vi "UIStep Execte UI Init.vi"(9 "Project Path":path, 10 "UI Setting":T1={"Embedded"=FALSE, "Size"=enum."Small", "Title"="", "Content"="", "Text Style"={"Font"="", "Size"=0.0, "Justification"=1, "TextColor"=0, "BGColor"=0, "Bold"=FALSE}, "Buttons"={"Button1"={"Label"="", "Size"=0.0, "TextColor"=0, "BGColor"=0, "Bold"=FALSE}, "Button2"={"Label"="", "Size"=0.0, "TextColor"=0, "BGColor"=0, "Bold"=FALSE}}, "Image"=path "", "Enable Input"=FALSE, "Input Validation"=""} {"Text Style"."Justification" items=["Left", "Center", "Right"]}, 11 "UI Control":T2) -> (3 "UI Control out":T2)   [LabVIEW 2015, in "UIStep.lvclass"]
uses:
  UIStep.lvclass
  <vilib>/Utility/miscctls.llb/LVPointTypeDef.ctl
  <vilib>/Utility/miscctls.llb/LVRectTypeDef.ctl
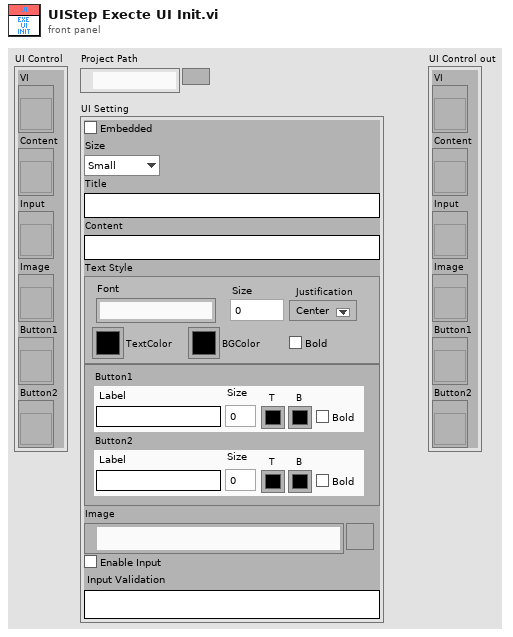
[diagram p1: front panel]
types:
  T1 = cluster{"Embedded":bool, "Size":enum16{"Small", "Middle", "Big"}, "Title":string, "Content":string, "Text Style":cluster{"Font":string, "Size":dbl, "Justification":u16, "TextColor":u32, "BGColor":u32, "Bold":bool}, "Buttons":cluster{"Button1":cluster{"Label":string, "Size":dbl, "TextColor":u32, "BGColor":u32, "Bold":bool}, "Button2":cluster{"Label":string, "Size":dbl, "TextColor":u32, "BGColor":u32, "Bold":bool}}, "Image":path, "Enable Input":bool, "Input Validation":string}
  T2 = cluster{"VI":refnum<vi>, "Content":refnum<vi>, "Input":refnum<vi>, "Image":refnum<vi>, "Button1":refnum<vi>, "Button2":refnum<vi>}
  T3 = typedef "LVPointTypeDef.ctl" = cluster{"Horizontal":i16, "Vertical":i16}
  T4 = cluster{"Label":string, "Size":dbl, "TextColor":u32, "BGColor":u32, "Bold":bool}
  T5 = cluster{"Font":string, "Size":dbl, "Justification":u16, "TextColor":u32, "BGColor":u32, "Bold":bool}
  T6 = typedef "imagedata.ctl" = cluster{"image type":i32, "image depth":i32, "image":u8[], "mask":u8[], "colors":u32[], "Rectangle":cluster{"left":i16, "top":i16, "right":i16, "bottom":i16}}
  T7 = typedef "LVRectTypeDef.ctl" = cluster{"Left":i16, "Top":i16, "Right":i16, "Bottom":i16}
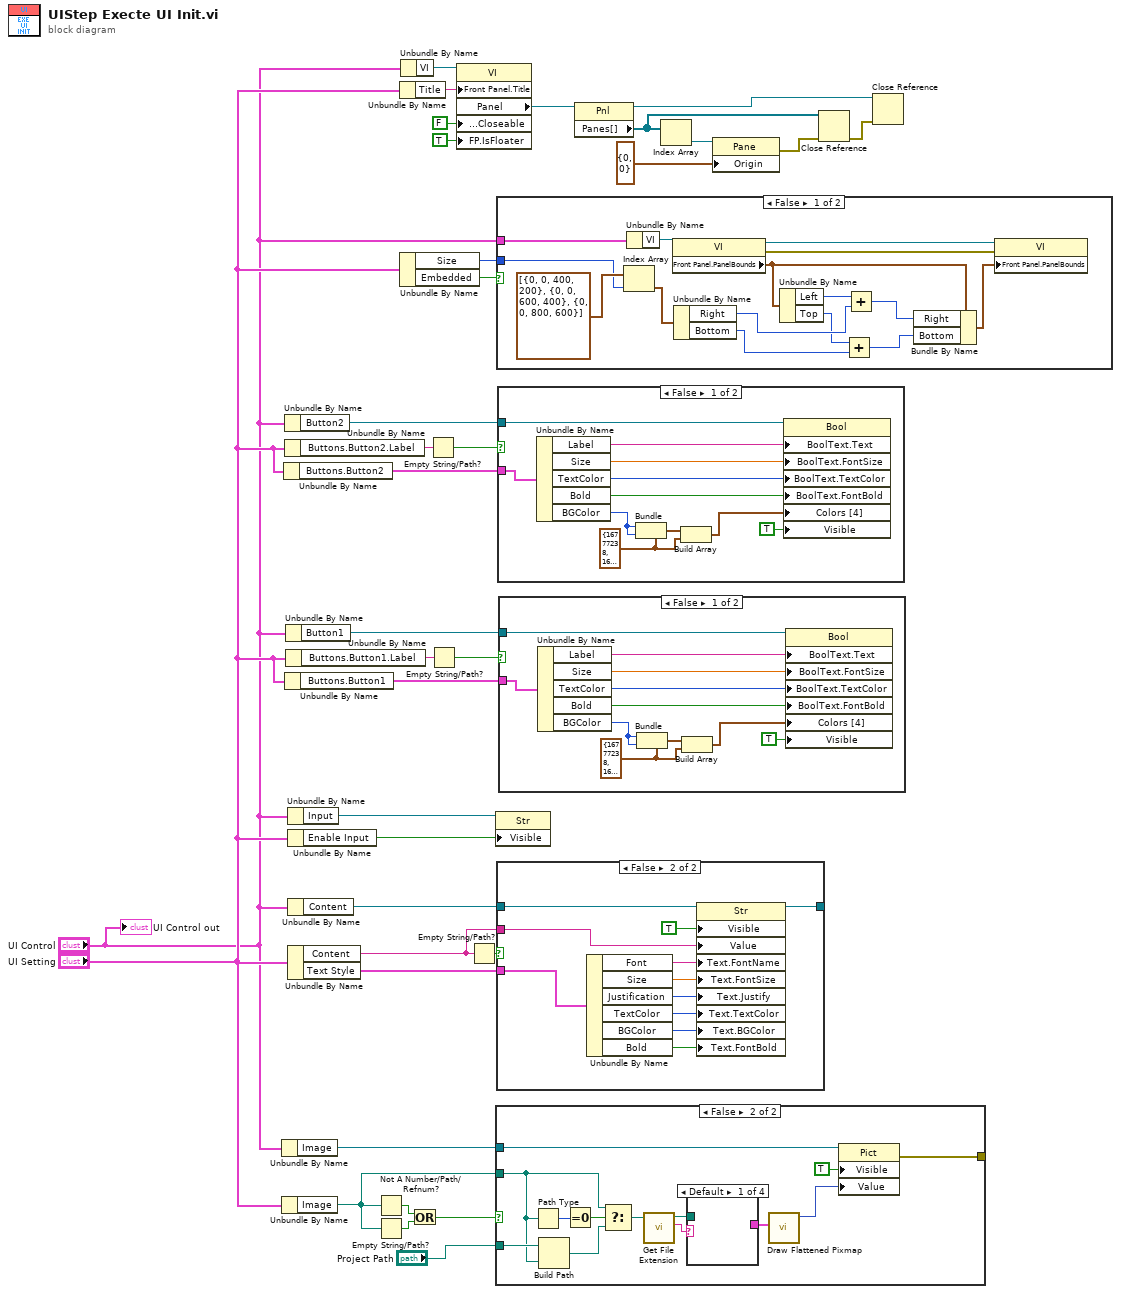
[diagram p0: block diagram]
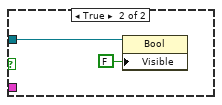
[diagram p3: hidden frame]
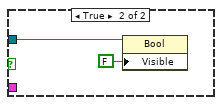
[diagram p4: hidden frame]
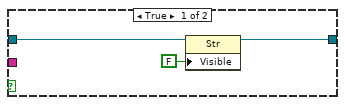
[diagram p5: hidden frame]
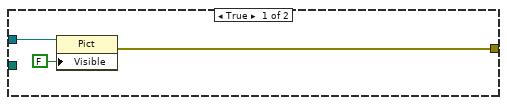
[diagram p6: hidden frame]
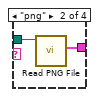
[diagram p7: hidden frame]
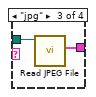
[diagram p8: hidden frame]
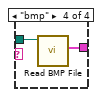
[diagram p9: hidden frame]
diagram:
  n1 = Unbundle By Name("UI Control") -> ("Image"=w35:refnum<vi>)
  n2 = Unbundle By Name("UI Setting") -> ("Image"=w31:path)
  n3 = Unbundle By Name("UI Setting") -> ("Buttons.Button2"=w20:T4)
  n4 = Unbundle By Name("UI Control") -> ("Button2"=w19:refnum<vi>)
  n5 = Unbundle By Name("UI Setting") -> ("Buttons.Button2.Label"=w17:string)
  n6 = Unbundle By Name("UI Setting") -> ("Buttons.Button1"=w21:T4)
  n7 = Unbundle By Name("UI Control") -> ("Button1"=w22:refnum<vi>)
  n8 = Unbundle By Name("UI Setting") -> ("Buttons.Button1.Label"=w24:string)
  n9 = Unbundle By Name("UI Control") -> ("Input"=w25:refnum<vi>)
  n10 = Unbundle By Name("UI Setting") -> ("Enable Input"=w3:bool)
  n11 = Unbundle By Name("UI Control") -> ("Content"=w28:refnum<vi>)
  n12 = Unbundle By Name("UI Setting") -> ("Content"=w26:string, "Text Style"=w27:T5)
  n13 = Not A Number/Path/Refnum?(number/path/refnum=w31) -> (NaN/Path/Refnum?=w33:bool)
  n14 = Empty String/Path?(string/path=w31) -> (empty?=w34:bool)
  n15 = Unbundle By Name("UI Setting") -> ("Title"=w15:string)
  n16 = Unbundle By Name("UI Setting") -> ("Size"=w6:enum16{"Small", "Middle", "Big"}, "Embedded"=w7:bool)
  n17 = Unbundle By Name("UI Control") -> ("VI"=w16:refnum<vi>)
  n18 = Or(x=w33, y=w34) -> (x .or. y?=w32:bool)
  n19 = Empty String/Path?(string/path=w17) -> (empty?=w18:bool)
  n20 = Empty String/Path?(string/path=w24) -> (empty?=w23:bool)
  n21 = property class="VI"(reference=w16, "Front Panel.Title"=w15, "Front Panel.Closeable"=FALSE ("Front Panel Window:Closeable"), "FP.IsFloater"=TRUE ("Front Panel Window:Is Floating")) -> ("Panel"=w14:refnum<vi>)  [unwired: 1 in, 2 out]
  n22 = Empty String/Path?(string/path=w26) -> (empty?=w29:bool)
  n23 = property class="Str"(reference=w25, "Visible"=w3) -> ()  [unwired: 1 in, 2 out]
  n24 = case shown="False" w32 {
    tunnel: w35 -> [w38 w51]
    tunnel: w31 -> [_ w46]
    tunnel: "Project Path" -> [_ w47]
    tunnel: [w36 w42] -> _
    frame True {
      n25 = property class="Pict"(reference=w38, "Visible"=FALSE) -> (error out=w36:errorcluster)  [unwired: 1 in, 1 out]
    }
    frame False {
      n26 = Path Type(1:w46) -> (0:w49:i16)
      n27 = Build Path(base path=w47, name or relative path=w46) -> (appended path=w45:path)
      n28 = Equal To 0?(x=w49) -> (x = 0?=w48:bool)
      n29 = Select(t=w46, s=w48, f=w45) -> (s? t:f=w41:path)
      n30 = call <vilib>:"Get File Extension.vi"("file"=w41) -> ("lowercase file extension"=w39:string, "dup file"=w40:path)  [unwired: 6 in, 3 out]
      n31 = case shown="Default" w39 {
        tunnel: [_ w53 w55 w57] -> w44
        tunnel: w40 -> [_ w52 w54 w56]
        frame Default {
        }
        frame "png" {
          n32 = call <vilib>:"Read PNG File.vi"("path to PNG file"=w52) -> ("image data"=w53:T6)  [unwired: 8 in, 2 out]
        }
        frame "jpg" {
          n33 = call <vilib>:"Read JPEG File.vi"("path to JPEG file"=w54) -> ("image data"=w55:T6)  [unwired: 8 in, 2 out]
        }
        frame "bmp" {
          n34 = call <vilib>:"Read BMP File.vi"("path to BMP file"=w56) -> ("image data"=w57:T6)  [unwired: 8 in, 2 out]
        }
      }
      n35 = call <vilib>:"Draw Flattened Pixmap.vi"("image data"=w44) -> ("new picture"=w43:picture)  [unwired: 8 in]
      n36 = property class="Pict"(reference=w51, "Visible"=TRUE, "Value"=w43) -> (error out=w42:errorcluster)  [unwired: 1 in, 1 out]
    }
  }
  n37 = case shown="False" w7 {
    tunnel: "UI Control" -> [w71 _]
    tunnel: w6 -> [w69 _]
    frame False {
      n38 = Index Array(array=T7[] [{"Left"=0, "Top"=0, "Right"=400, "Bottom"=200}, {"Left"=0, "Top"=0, "Right"=600, "Bottom"=400}, {"Left"=0, "Top"=0, "Right"=800, "Bottom"=600}], index=w69) -> (element=w66:T7)
      n39 = Unbundle By Name(w71) -> ("VI"=w72:refnum<vi>)
      n40 = property class="VI"(reference=w72) -> (reference out=w68:refnum<vi>, error out=w67:errorcluster, "Front Panel.PanelBounds"=w65:T7)  [unwired: 1 in]
      n41 = Unbundle By Name(w66) -> ("Right"=w62:i16, "Bottom"=w59:i16)
      n42 = Unbundle By Name(w65) -> ("Left"=w63:i16, "Top"=w60:i16)
      n43 = Add(x=w60, y=w59) -> (x+y=w58:i16)
      n44 = Add(x=w63, y=w62) -> (x+y=w61:i16)
      n45 = Bundle By Name(cluster=w65, "Right"=w61, "Bottom"=w58) -> (w64:T7)
      n46 = property class="VI"(reference=w68, error in=w67, "Front Panel.PanelBounds"=w64) -> ()  [unwired: 2 out]
    }
    frame True {
    }
  }
  n47 = case shown="False" w29 {
    tunnel: w28 -> [w75 w86]
    tunnel: w27 -> [_ w84]
    tunnel: w26 -> [_ w83]
    tunnel: [w73 w76] -> _
    frame True {
      n48 = property class="Str"(reference=w75, "Visible"=FALSE) -> (reference out=w73:refnum<vi>)  [unwired: 1 in, 1 out]
    }
    frame False {
      n49 = Unbundle By Name(w84) -> ("Font"=w82:string, "Size"=w81:dbl, "Justification"=w80:u16, "TextColor"=w79:u32, "BGColor"=w78:u32, "Bold"=w77:bool)
      n50 = property class="Str"(reference=w86, "Visible"=TRUE, "Value"=w83, "Text.FontName"=w82, "Text.FontSize"=w81, "Text.Justify"=w80, "Text.TextColor"=w79, "Text.BGColor"=w78, "Text.FontBold"=w77) -> (reference out=w76:refnum<vi>)  [unwired: 1 in, 1 out]
    }
  }
  n51 = case shown="False" w18 {
    tunnel: w19 -> [w97 w99]
    tunnel: w20 -> [w96 _]
    frame False {
      w89 = cluster{u32, u32} {16777238, 16777238}
      n52 = Unbundle By Name(w96) -> ("Label"=w95:string, "Size"=w94:dbl, "TextColor"=w93:u32, "Bold"=w92:bool, "BGColor"=w91:u32)
      n53 = Bundle(cluster=w89, w91, w91) -> (w90:cluster{u32, u32})
      n54 = Build Array(w90, w89) -> (w88:cluster{u32, u32}[])
      n55 = property class="Bool"(reference=w97, "BoolText.Text"=w95, "BoolText.FontSize"=w94, "BoolText.TextColor"=w93, "BoolText.FontBold"=w92, "Colors [4]"=w88, "Visible"=TRUE) -> ()  [unwired: 1 in, 2 out]
    }
    frame True {
      n56 = property class="Bool"(reference=w99, "Visible"=FALSE) -> ()  [unwired: 1 in, 2 out]
    }
  }
  n57 = case shown="False" w23 {
    tunnel: w22 -> [w110 w112]
    tunnel: w21 -> [w109 _]
    frame False {
      w102 = cluster{u32, u32} {16777238, 16777238}
      n58 = Unbundle By Name(w109) -> ("Label"=w108:string, "Size"=w107:dbl, "TextColor"=w106:u32, "Bold"=w105:bool, "BGColor"=w104:u32)
      n59 = Bundle(cluster=w102, w104, w104) -> (w103:cluster{u32, u32})
      n60 = Build Array(w103, w102) -> (w101:cluster{u32, u32}[])
      n61 = property class="Bool"(reference=w110, "BoolText.Text"=w108, "BoolText.FontSize"=w107, "BoolText.TextColor"=w106, "BoolText.FontBold"=w105, "Colors [4]"=w101, "Visible"=TRUE) -> ()  [unwired: 1 in, 2 out]
    }
    frame True {
      n62 = property class="Bool"(reference=w112, "Visible"=FALSE) -> ()  [unwired: 1 in, 2 out]
    }
  }
  n63 = property class="Pnl"(reference=w14) -> (reference out=w8:refnum<vi>, "Panes[]"=w10:refnum<vi>[])  [unwired: 1 in, 1 out]
  n64 = Index Array(array=w10) -> (element=w13:refnum<vi>)  [unwired: 1 in]
  n65 = property class="Pane"(reference=w13, "Origin"=T3 {"Horizontal"=0, "Vertical"=0}) -> (error out=w11:errorcluster)  [unwired: 1 in, 1 out]
  n66 = Close Reference(reference=w10, error in (no error)=w11) -> (error out=w9:errorcluster)
  n67 = Close Reference(reference=w8, error in (no error)=w9) -> ()  [unwired: 1 out]
  "UI Control out" <- "UI Control"
